vi "count.trues.vi"(11 "enabled":bool[](array[boolean])=[FALSE, FALSE, FALSE, FALSE, FALSE, FALSE, FALSE, FALSE]) -> (3 "Numeric":u8)   [LabVIEW 2022 SP3]
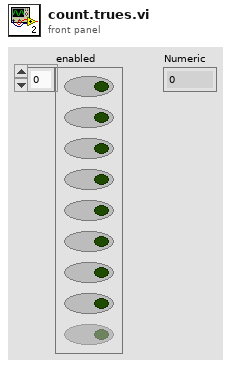
[diagram p1: front panel]
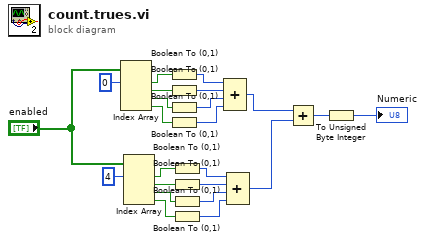
[diagram p0: block diagram]
diagram:
  n1 = Index Array(array="enabled", index #1=0 ("index")) -> (element #1=w3:bool, element #2=w5:bool, element #3=w7:bool, element #4=w10:bool)  [unwired: 3 in]
  n2 = Index Array(array="enabled", index #1=4 ("index")) -> (element #1=w13:bool, element #2=w15:bool, element #3=w17:bool, element #4=w20:bool)  [unwired: 3 in]
  n3 = Boolean To (0,1)(Boolean=w3) -> (0, 1=w4:i16)
  n4 = Boolean To (0,1)(Boolean=w5) -> (0, 1=w6:i16)
  n5 = Boolean To (0,1)(Boolean=w7) -> (0, 1=w8:i16)
  n6 = Boolean To (0,1)(Boolean=w10) -> (0, 1=w9:i16)
  n7 = Boolean To (0,1)(Boolean=w13) -> (0, 1=w14:i16)
  n8 = Boolean To (0,1)(Boolean=w15) -> (0, 1=w16:i16)
  n9 = Boolean To (0,1)(Boolean=w17) -> (0, 1=w18:i16)
  n10 = Boolean To (0,1)(Boolean=w20) -> (0, 1=w19:i16)
  n11 = Compound Arithmetic op=ADD(w4, w6, w8, w9) -> (w11:i16)
  n12 = Compound Arithmetic op=ADD(w14, w16, w18, w19) -> (w22:i16)
  n13 = Add(x=w11, y=w22) -> (x+y=w23:i16)
  n14 = To Unsigned Byte Integer(number=w23) -> (unsigned 8bit integer=→"Numeric":u8)
